vi "Rx 2945 2955 Aurora.vi"(0 "rx.parameters":T3={"rx.trigger select"=enum."Software", "rx.trigger enable"=FALSE, "rx.trigger sync enable"=FALSE, "rx.stream enable"=[FALSE, FALSE, FALSE, FALSE], "rx.software trigger"=FALSE, "rx.reset"=FALSE, "rx.abort"=FALSE, "rx.samples to acquire"=0, "rx.data sink"=enum."SFP Port 0", "rx.ddc parameters"=[{"output sample rate"=0.0, "delay"=0.0, "frequency shift"=0.0, "impairments"={"inline gain I"=0.0, "inline gain Q"=0.0, "cross gain I"=0.0, "cross gain Q"=0.0, "pre-gain offset I"=0.0, "pre-gain offset Q"=0.0, "post-gain offset I"=0.0, "post-gain offset Q"=0.0}, "phase"=0.0}, {"output sample rate"=0.0, "delay"=0.0, "frequency shift"=0.0, "impairments"={"inline gain I"=0.0, "inline gain Q"=0.0, "cross gain I"=0.0, "cross gain Q"=0.0, "pre-gain offset I"=0.0, "pre-gain offset Q"=0.0, "post-gain offset I"=0.0, "post-gain offset Q"=0.0}, "phase"=0.0}, {"output sample rate"=0.0, "delay"=0.0, "frequency shift"=0.0, "impairments"={"inline gain I"=0.0, "inline gain Q"=0.0, "cross gain I"=0.0, "cross gain Q"=0.0, "pre-gain offset I"=0.0, "pre-gain offset Q"=0.0, "post-gain offset I"=0.0, "post-gain offset Q"=0.0}, "phase"=0.0}, {"output sample rate"=0.0, "delay"=0.0, "frequency shift"=0.0, "impairments"={"inline gain I"=0.0, "inline gain Q"=0.0, "cross gain I"=0.0, "cross gain Q"=0.0, "pre-gain offset I"=0.0, "pre-gain offset Q"=0.0, "post-gain offset I"=0.0, "post-gain offset Q"=0.0}, "phase"=0.0}]} {"rx.ddc parameters"."frequency shift" format="%#.48g"}, 1 "Simulate Data":bool, 5 "rx.start trigger":bool) -> (4 "rx.status":T2={"rx.state"=enum."Idle", "rx.samples processed"=0, "rx.number of fifo overflows"=0, "rx.number of iq data overflows"=[0, 0, 0, 0], "rx.dsp reset done"=FALSE})   [LabVIEW 2016]
uses:
  Rx Parameters.ctl
  HOST/29x5/SubVIs/Start Trigger.ctl
  DDC Parameters.ctl
  <instrlib>/_niInstr/DSP/v1/Shared/Public/IQ Impairments.ctl
  Stream Control State.ctl
  <instrlib>/_niInstr/DSP/v1/Shared/niInstr DSP v1 Shared.lvlib
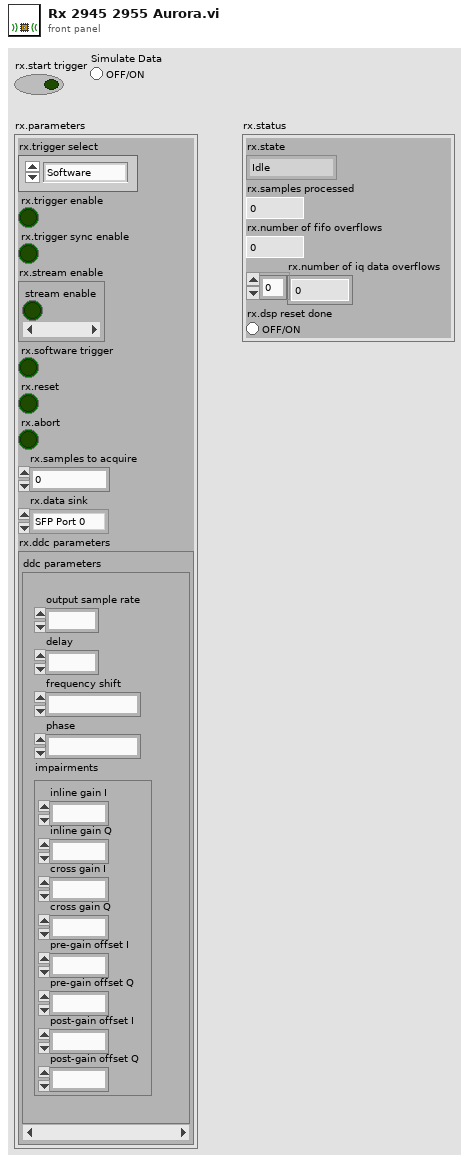
[diagram p1: front panel]
types:
  T1 = typedef "Stream Control State.ctl" = enum16{"Idle", "Active"}
  T2 = cluster{"rx.state":T1, "rx.samples processed":u32, "rx.number of fifo overflows":u32, "rx.number of iq data overflows":u64[], "rx.dsp reset done":bool}
  T3 = typedef "Rx Parameters.ctl" = cluster{"rx.trigger select":T4, "rx.trigger enable":bool, "rx.trigger sync enable":bool, "rx.stream enable":bool[], "rx.software trigger":bool, "rx.reset":bool, "rx.abort":bool, "rx.samples to acquire":u32, "rx.data sink":enum16{"SFP Port 0", "SFP Port 1", "Host"}, "rx.ddc parameters":T5[]}
  T4 = typedef "Start Trigger.ctl" = enum8{"Software", "Digital Edge", "Rx Start Trigger", "Tx Start Trigger", "Immediate", "Future Time Event"}
  T5 = typedef "DDC Parameters.ctl" = cluster{"output sample rate":fxp<+,48,1>, "delay":fxp<+/-,16,0>, "frequency shift":fxp<+/-,48,0>, "impairments":T6, "phase":fxp<+/-,21,0>}
  T6 = typedef "niInstr DSP v1 Shared.lvlib/IQ Impairments.ctl" = cluster{"inline gain I":fxp<+/-,18,1>, "inline gain Q":fxp<+/-,18,1>, "cross gain I":fxp<+/-,18,1>, "cross gain Q":fxp<+/-,18,1>, "pre-gain offset I":fxp<+/-,18,1>, "pre-gain offset Q":fxp<+/-,18,1>, "post-gain offset I":fxp<+/-,18,1>, "post-gain offset Q":fxp<+/-,18,1>}
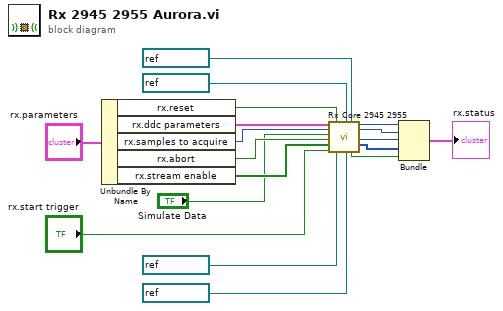
[diagram p0: block diagram]
diagram:
  n1 = Unbundle By Name("rx.parameters") -> ("rx.reset"=w14:bool, "rx.ddc parameters"=w17:T5[], "rx.samples to acquire"=w16:u32, "rx.abort"=w15:bool, "rx.stream enable"=w6:bool[])
  n2 = call "Rx Core 2945 2955.vi"("rx.ddc parameters"=w17, "rx.samples to acquire"=w16, "Simulate Data"="Simulate Data", "rx.abort"=w15, "rx.stream enable"=w6, "rx.start trigger"="rx.start trigger", "rx.reset"=w14, "fifo 2"=refnum<k21> "rx 2.fifo", "fifo 0"=refnum<k21> "rx 0.fifo", "fifo 3"=refnum<k21> "rx 3.fifo", "fifo 1"=refnum<k21> "rx 1.fifo") -> ("rx.dsp reset done"=w9:bool, "rx.state"=w12:T1, "rx.samples processed"=w11:u32, "rx.number of fifo overflows"=w10:u32, "rx.number of iq data overflows"=w5:u64[])  [unwired: 4 in]
  n3 = Bundle("rx.state"=w12, "rx.samples processed"=w11, "rx.number of fifo overflows"=w10, "rx.number of iq data overflows"=w5, "rx.dsp reset done"=w9) -> (→"rx.status":T2)  [unwired: 1 in]
